vi "sub_log_gnss.vi"(7 "cmd":enum16{"GNSS", "Scout"}(ring), 8 "error in":errorcluster, 11 "log_data":string) -> (0 "error out":errorcluster)   [LabVIEW 2019]
uses:
  Subvi/log/logfile-name.vi
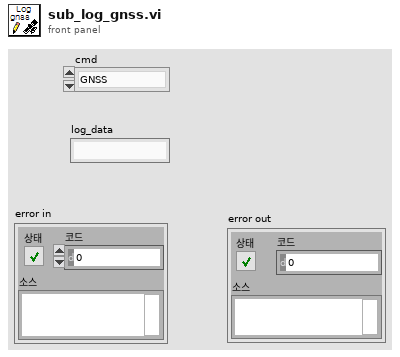
[diagram p1: front panel]
types:
  T1 = enum16{"open", "replace", "create", "open or create", "replace or create", "replace or create with confirmation"}
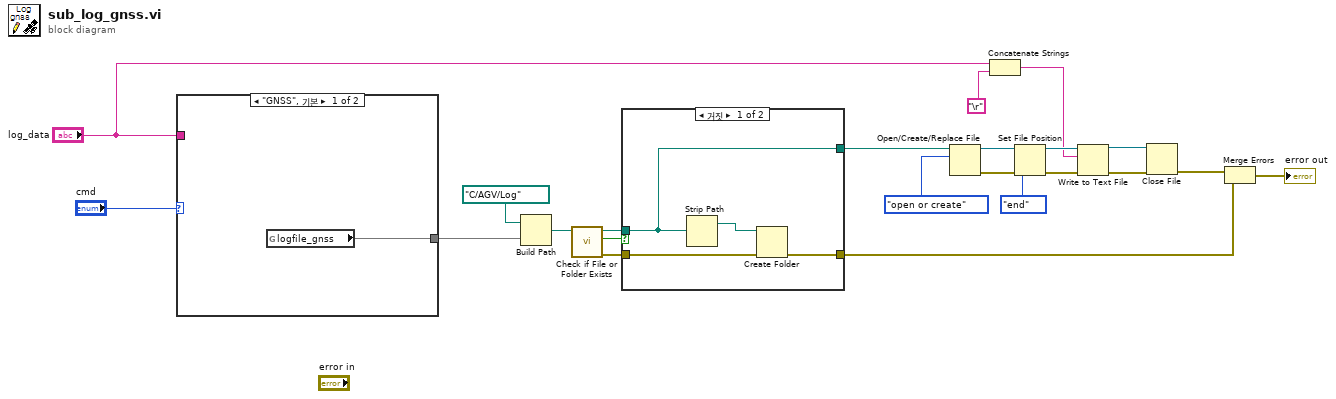
[diagram p0: block diagram]
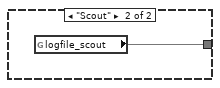
[diagram p2: hidden frame]
diagram:
  n1 = case shown="\"GNSS\", 기본" "cmd" {
    tunnel: [w23 w24] -> w3
    tunnel: "log_data" -> [_ _]
    frame "GNSS", Default {
      n2 = global read "logfile-name.vi" "logfile_gnss"() -> (w23)
    }
    frame "Scout" {
      n3 = global read "logfile-name.vi" "logfile_scout"() -> (w24)
    }
  }
  n4 = Build Path(base path=path "C:/AGV/Log" ("베이스 경로"), name or relative path=w3) -> (appended path=w9:path)
  n5 = call <vilib>:"Check if File or Folder Exists.vi"("path"=w9) -> ("error out"=w5:errorcluster, "file or folder exists?"=w10:bool, "dup path"=w21:path)  [unwired: 8 in]
  n6 = case shown="거짓" w10 {
    tunnel: w21 -> [w27 w30]
    tunnel: [w27 w30] -> w8
    tunnel: [w26 w29] -> w6
    tunnel: w5 -> [w25 w29]
    frame False {
      n7 = Strip Path(path=w27) -> (stripped path=w28:path)  [unwired: 1 out]
      n8 = Create Folder(path (use dialog)=w28, error in=w25) -> (error out=w26:errorcluster)  [unwired: 1 in, 2 out]
    }
    frame True {
    }
  }
  n9 = Open/Create/Replace File(file path (use dialog)=w8, operation (0:open)=T1."open or create" ("동작(0:open)")) -> (refnum out=w18:refnum<file>, error out=w17:errorcluster)  [unwired: 4 in, 1 out]
  n10 = Concatenate Strings("log_data", "\r") -> (w11:string)
  n11 = Set File Position(refnum=w18, from (0:start)=enum16{"start", "end", "current"}."end" ("위치(0:start)"), error in=w17) -> (refnum out=w14:refnum<file>, error out=w15:errorcluster)  [unwired: 1 in]
  n12 = Write to Text File(file (use dialog)=w14, text=w11, error in=w15) -> (refnum out=w12:refnum<file>, error out=w13:errorcluster)  [unwired: 1 in, 1 out]
  n13 = Close File(refnum=w12, error in=w13) -> (error out=w7:errorcluster)  [unwired: 1 out]
  n14 = Merge Errors(w7, w6) -> (→"error out":errorcluster)
